vi "Init.vi"(8 "error in (no error)":errorcluster, 11 "UI Actor in":refnum<class "UI Actor.lvclass">) -> (0 "error out":errorcluster, 3 "UI Actor out":refnum<class "UI Actor.lvclass">)   [LabVIEW 2020, in "UI Actor.lvlib" / "UI Actor.lvclass"]
uses:
  UI Actor.lvclass
  C:/Program Files (x86)/National Instruments/LabVIEW 2020/vi.lib/ActorFramework/Actor/Actor.lvclass
  UI Actor.lvclass/UI Actor.ctl
  Coca Actors/Coca Actors.lvclass
  Coca Actors/Coca Actors.lvclass/Coca Actors.ctl
  Sabritas Actor/Sabritas Actor.lvclass
  Sabritas Actor/Sabritas Actor.lvclass/Sabritas Actor.ctl
  MXN Actor/MXN Actor.lvclass
  MXN Actor/MXN Actor.lvclass/MXN Actor.ctl
  USD Actor/USD Actor.lvclass
  USD Actor/USD Actor.lvclass/USD Actor.ctl
  ESP Actor/ESP Actor.lvclass
  ESP Actor/ESP Actor.lvclass/ESP Actor.ctl
  ENG Actor/ENG Actor.lvclass
  ENG Actor/ENG Actor.lvclass/ENG Actor.ctl
  Get Coins.vi
  Get Sub Panel Coins.vi
  Get Products.vi
  Get Sub Panel Prods.vi
  Get Language.vi
  Get Sub Panel Msg.vi
  <vilib>/ActorFramework/Actor/Actor.lvclass
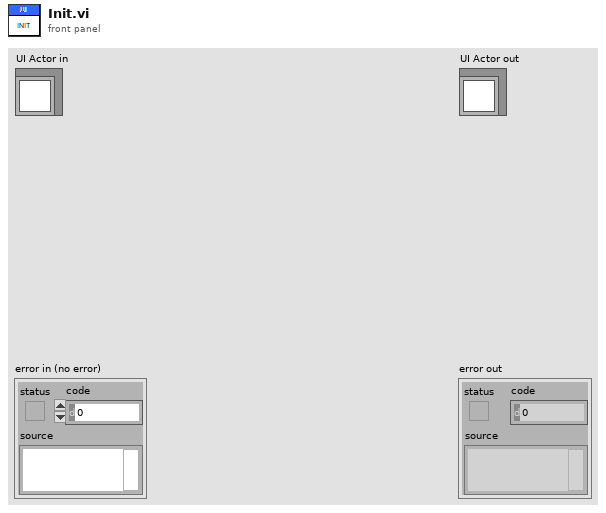
[diagram p1: front panel]
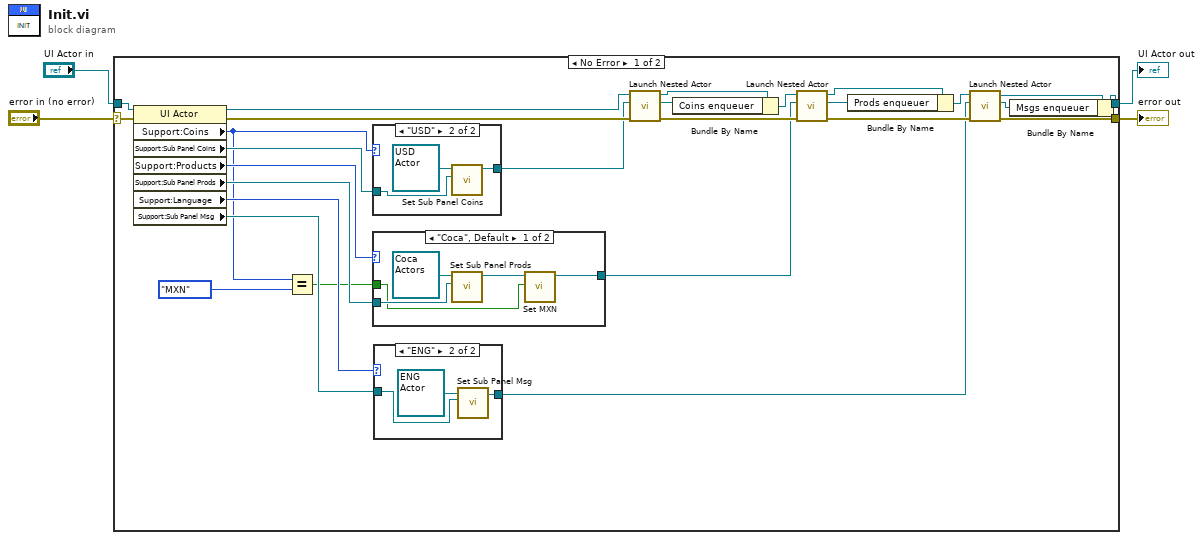
[diagram p0: block diagram]
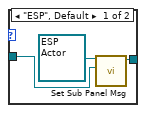
[diagram p2: hidden frame]
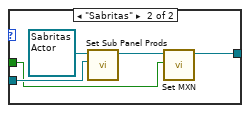
[diagram p3: hidden frame]
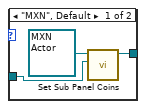
[diagram p4: hidden frame]
diagram:
  n1 = case shown="No Error" "error in (no error)" {
    selector: "error in (no error)" -> [w31 w55]
    tunnel: [w13 w55] -> w3
    tunnel: [w9 w54] -> w1
    tunnel: "UI Actor in" -> [w30 w54]
    frame No Error {
      n2 = property class="UI Actor"(reference=w30, error in=w31) -> (reference out=w21:refnum<class "UI Actor.lvclass">, error out=w23:errorcluster, "Support:Coins"=w7:enum16{"MXN", "USD"}, "Support:Sub Panel Coins"=w26:refnum<vi>, "Support:Products"=w25:enum16{"Coca", "Sabritas"}, "Support:Sub Panel Prods"=w24:refnum<vi>, "Support:Language"=w15:enum16{"ESP", "ENG"}, "Support:Sub Panel Msg"=w14:refnum<vi>)
      n3 = Equal?(x=w7, y=enum16{"MXN", "USD"}."MXN") -> (x = y?=w5:bool)
      n4 = case shown="\"USD\"" w7 {
        tunnel: [w49 w53] -> w18
        tunnel: w26 -> [w48 w51]
        frame "MXN", Default {
          n5 = call "Set Sub Panel Coins.vi"("Sub Panel Coins"=w48, "MXN Actor in"=refnum<class "MXN Actor.lvclass"> refnum ("MXN Actor.lvlib:MXN Actor.lvclass")) -> ("MXN Actor out"=w49:refnum<class "MXN Actor.lvclass">)  [unwired: 8 in, 1 out]
        }
        frame "USD" {
          n6 = call "Set Sub Panel Coins.vi"("Sub Panel Coins"=w51, "USD Actor in"=refnum<class "USD Actor.lvclass"> refnum ("USD Actor.lvlib:USD Actor.lvclass")) -> ("USD Actor out"=w53:refnum<class "USD Actor.lvclass">)  [unwired: 8 in, 1 out]
        }
      }
      n7 = case shown="\"Coca\", Default" w25 {
        tunnel: w24 -> [w41 w46]
        tunnel: [w39 w44] -> w17
        tunnel: w5 -> [w38 w43]
        frame "Coca", Default {
          n8 = call "Set Sub Panel Prods.vi"("Sub Panel Prods"=w41, "Coca Actors in"=refnum<class "Coca Actors.lvclass"> refnum ("Coca Actors.lvlib:Coca Actors.lvclass")) -> ("Coca Actors out"=w40:refnum<class "Coca Actors.lvclass">)  [unwired: 8 in, 1 out]
          n9 = call "Set MXN.vi"("MXN"=w38, "Coca Actors in"=w40) -> ("Coca Actors out"=w39:refnum<class "Coca Actors.lvclass">)  [unwired: 8 in, 1 out]
        }
        frame "Sabritas" {
          n10 = call "Set Sub Panel Prods.vi"("Sub Panel Prods"=w46, "Sabritas Actor in"=refnum<class "Sabritas Actor.lvclass"> refnum ("Sabritas Actor.lvlib:Sabritas Actor.lvclass")) -> ("Sabritas Actor out"=w45:refnum<class "Sabritas Actor.lvclass">)  [unwired: 8 in, 1 out]
          n11 = call "Set MXN.vi"("MXN"=w43, "Sabritas Actor in"=w45) -> ("Sabritas Actor out"=w44:refnum<class "Sabritas Actor.lvclass">)  [unwired: 8 in, 1 out]
        }
      }
      n12 = case shown="\"ENG\"" w15 {
        tunnel: w14 -> [w33 w35]
        tunnel: [w32 w36] -> w10
        frame "ESP", Default {
          n13 = call "Set Sub Panel Msg.vi"("Sub Panel Msg"=w33, "ESP Actor in"=refnum<class "ESP Actor.lvclass"> refnum ("ESP Actor.lvlib:ESP Actor.lvclass")) -> ("ESP Actor out"=w32:refnum<class "ESP Actor.lvclass">)  [unwired: 8 in, 1 out]
        }
        frame "ENG" {
          n14 = call "Set Sub Panel Msg.vi"("Sub Panel Msg"=w35, "ENG Actor in"=refnum<class "ENG Actor.lvclass"> refnum ("ENG Actor.lvlib:ENG Actor.lvclass")) -> ("ENG Actor out"=w36:refnum<class "ENG Actor.lvclass">)  [unwired: 8 in, 1 out]
        }
      }
      n15 = call <vilib>:"Launch Nested Actor.vi"("error in (no error)"=w23, "Nested Actor"=w18, "Caller Actor in"=w21) -> ("error out"=w22:errorcluster, "Nested Actor's Enqueuer"=w16:refnum<class "Message Enqueuer.lvclass">, "Caller Actor out"=w20:refnum<class "UI Actor.lvclass">)  [unwired: 6 in]
      n16 = Bundle By Name(cluster=w20, "Coins enqueuer"=w16) -> (w19:refnum<class "UI Actor.lvclass">)
      n17 = call <vilib>:"Launch Nested Actor.vi"("error in (no error)"=w22, "Nested Actor"=w17, "Caller Actor in"=w19) -> ("error out"=w29:errorcluster, "Nested Actor's Enqueuer"=w27:refnum<class "Message Enqueuer.lvclass">, "Caller Actor out"=w28:refnum<class "UI Actor.lvclass">)  [unwired: 6 in]
      n18 = Bundle By Name(cluster=w28, "Prods enqueuer"=w27) -> (w12:refnum<class "UI Actor.lvclass">)
      n19 = call <vilib>:"Launch Nested Actor.vi"("error in (no error)"=w29, "Nested Actor"=w10, "Caller Actor in"=w12) -> ("error out"=w13:errorcluster, "Nested Actor's Enqueuer"=w8:refnum<class "Message Enqueuer.lvclass">, "Caller Actor out"=w11:refnum<class "UI Actor.lvclass">)  [unwired: 6 in]
      n20 = Bundle By Name(cluster=w11, "Msgs enqueuer"=w8) -> (w9:refnum<class "UI Actor.lvclass">)
    }
    frame Error {
    }
  }
  "error out" <- w3
  "UI Actor out" <- w1
